vi "ResonatorModulation.vi"(8 "Initial Resonator Voltage":dbl=3.2590378278493897, 9 "Threshold (MHz)":dbl=0.1, 10 "Initial Slow Resonator Voltage":dbl, 11 "f_actual":dbl=394443079.9163828 format="%#_14f") -> (0 "error out":errorcluster, 1 "Slow Resonator Voltage":dbl, 3 "Fast Resonator Voltage":dbl=6.2440401279926325)   [LabVIEW 2017]
uses:
  wlmData.dll
  <vilib>/Analysis/NI_AALBase.lvlib
  <vilib>/Analysis/baseanly.llb/Mean (DBL).vi
  Global M2.vi
panel:
  in  "NUmber Loops":i32=20
  in  "millisecond multiple":u32=1
  in  "DaQ 2":refnum<k21>="M2 Slow Resonator Mod"
  in  "PID gains":T1={"proportional gain (Kc)"=0.05, "integral time (Ti, s)"=0.005, "derivative time (Td, s)"=0.0}
  in  "stop":bool
  in  "DaQ":refnum<k21>="Voltage to M2 Resonator mod"
  out "df/MHz":dbl(graph)=-6.680025041103363
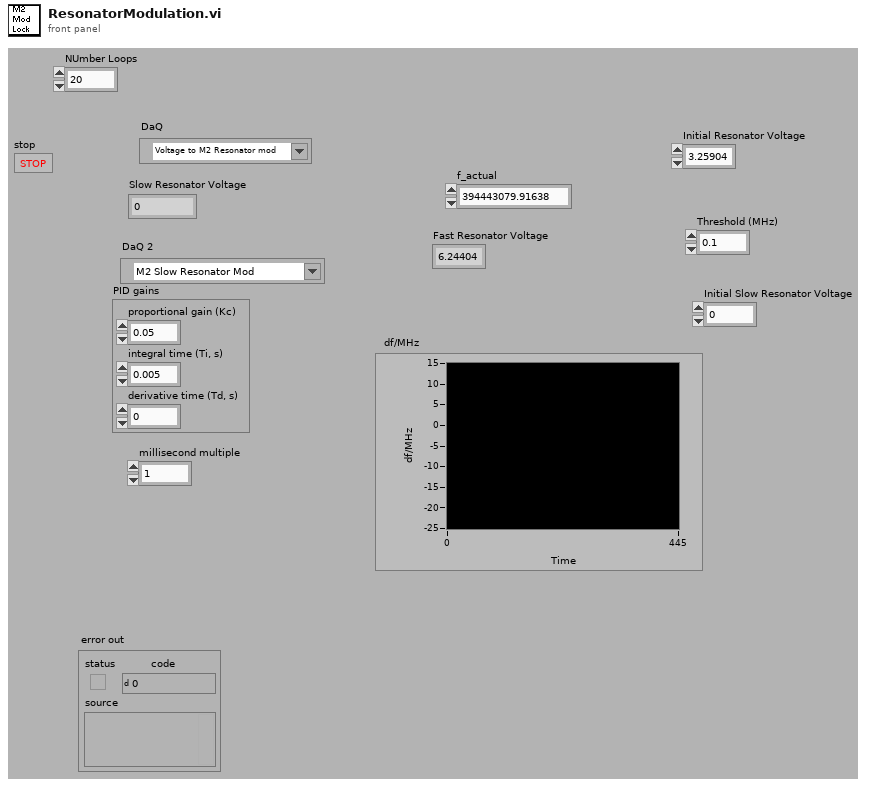
[diagram p1: front panel]
types:
  T1 = cluster{"proportional gain (Kc)":dbl, "integral time (Ti, s)":dbl, "derivative time (Td, s)":dbl}
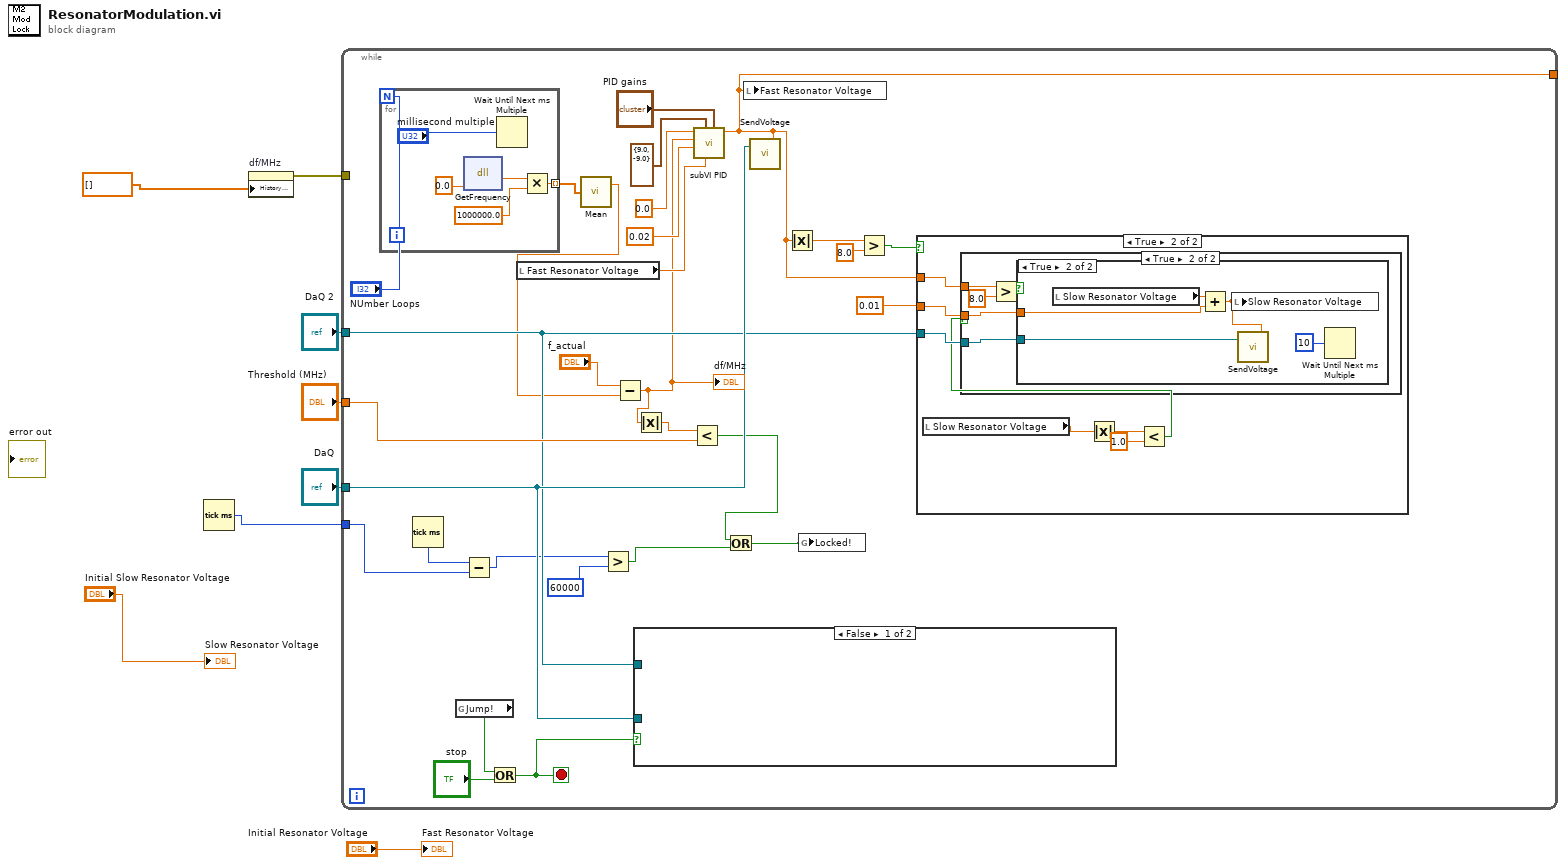
[diagram p0: block diagram]
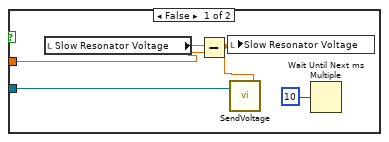
[diagram p4: hidden frame]
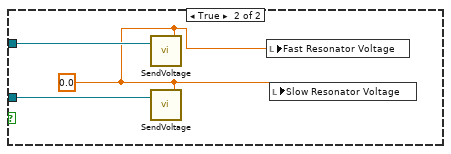
[diagram p5: hidden frame]
diagram:
  n1 = Tick Count (ms)() -> (millisecond timer value=w3:u32)
  n2 = property on="df/MHz" class="WFChart (strict)"("History Data"=dbl[] []) -> (error out=w1:errorcluster)  [unwired: 2 in, 1 out]
  n3 = while {
    tunnel: "DaQ" -> [w32]
    tunnel: [w22] -> _
    tunnel: "DaQ 2" -> [w29]
    tunnel: "Threshold (MHz)" -> [w30]
    tunnel: w3 -> [w20]
    tunnel: w1 -> [_]
    stop <- w27 stop-if-true
    n4 = for {
      N: "NUmber Loops" -> [_]
      tunnel: [w39] -> w14 mode=indexing
      n5 = dll-call lib="wlmData.dll" fn="GetFrequency"("arg1"=0.0) -> ("return type"=w41:dbl)  [unwired: 4 in, 2 out]
      n6 = Wait Until Next ms Multiple(millisecond multiple="millisecond multiple") -> ()  [unwired: 1 out]
      n7 = Multiply(x=w41, y=1000000.0) -> (x*y=w39:dbl)
    }
    n8 = Tick Count (ms)() -> (millisecond timer value=w21:u32)
    n9 = global read "Global M2.vi" "Jump!"() -> (w10:bool)
    n10 = Subtract(x=w21, y=w20) -> (x-y=w19:u32)
    n11 = Or(x=w10, y="stop") -> (x .or. y?=w27:bool)
    n12 = local read "Fast Resonator Voltage"() -> (w31:dbl)
    n13 = call-poly <vilib>:"Mean.vi"("X"=w14) -> ("mean"=w13:dbl)  [unwired: 1 out]
    n14 = Greater?(x=w19, y=u32 60000) -> (0:w17:bool)
    n15 = Subtract(x="f_actual", y=w13) -> (x-y=w12:dbl)
    "df/MHz" <- w12
    n16 = case shown="False" w27 {
      tunnel: w32 -> [_ w67]
      tunnel: w29 -> [_ w66]
      frame False {
      }
      frame True {
        w65 = sgl 0.0 ("value")
        n17 = call "SendVoltage.vi"("value"=w65, "DAQmx Global Channel"=w66) -> ()  [unwired: 1 in, 1 out]
        n18 = call "SendVoltage.vi"("value"=w65, "DAQmx Global Channel"=w67) -> ()  [unwired: 1 in, 1 out]
        n19 = local write "Fast Resonator Voltage"(w65) -> ()
        n20 = local write "Slow Resonator Voltage"(w65) -> ()
      }
    }
    n21 = Absolute Value(x=w12) -> (abs(x)=w11:dbl)
    n22 = Less?(x=w11, y=w30) -> (x < y?=w16:bool)
    n23 = call "subVI PID.vi"("PID gains"="PID gains", "input"=w31, "output range"=cluster{"output high":dbl, "output low":dbl} {"output high"=9.0, "output low"=-9.0}, "dt (s)"=0.02, "process variable"=w12, "setpoint"=0.0) -> ("output"=w22:dbl)  [unwired: 1 in, 4 out]
    n24 = Or(x=w16, y=w17) -> (x .or. y?=w9:bool)
    n25 = local write "Fast Resonator Voltage"(w22) -> ()
    n26 = call "SendVoltage.vi"("value"=w22, "DAQmx Global Channel"=w32) -> ()  [unwired: 1 in, 1 out]
    n27 = Absolute Value(x=w22) -> (abs(x)=w26:dbl)
    n28 = global write "Global M2.vi" "Locked!"(w9) -> ()
    n29 = Greater?(x=w26, y=8.0) -> (0:w24:bool)
    n30 = case shown="True" w24 {
      tunnel: w22 -> [_ w49]
      tunnel: w29 -> [_ w48]
      tunnel: 0.01 ("y") -> [_ w47]
      frame False {
      }
      frame True {
        n31 = local read "Slow Resonator Voltage"() -> (w46:dbl)
        n32 = Absolute Value(x=w46) -> (abs(x)=w45:dbl)
        n33 = Less?(x=w45, y=1.0) -> (x < y?=w43:bool)
        n34 = case shown="True" w43 {
          tunnel: w49 -> [_ w54]
          tunnel: w48 -> [_ w51]
          tunnel: w47 -> [_ w50]
          frame False {
          }
          frame True {
            n35 = Greater?(x=w54, y=8.0) -> (0:w52:bool)
            n36 = case shown="True" w52 {
              tunnel: w51 -> [w59 w63]
              tunnel: w50 -> [w56 w61]
              frame False {
                n37 = local read "Slow Resonator Voltage"() -> (w57:dbl)
                n38 = Subtract(x=w57, y=w56) -> (x-y=w55:dbl)
                n39 = local write "Slow Resonator Voltage"(w55) -> ()
                n40 = call "SendVoltage.vi"("value"=w55, "DAQmx Global Channel"=w59) -> ()  [unwired: 1 in, 1 out]
                n41 = Wait Until Next ms Multiple(millisecond multiple=u32 10) -> ()  [unwired: 1 out]
              }
              frame True {
                n42 = local read "Slow Resonator Voltage"() -> (w64:dbl)
                n43 = Add(x=w64, y=w61) -> (x+y=w62:dbl)
                n44 = local write "Slow Resonator Voltage"(w62) -> ()
                n45 = call "SendVoltage.vi"("value"=w62, "DAQmx Global Channel"=w63) -> ()  [unwired: 1 in, 1 out]
                n46 = Wait Until Next ms Multiple(millisecond multiple=u32 10) -> ()  [unwired: 1 out]
              }
            }
          }
        }
      }
    }
  }
  "Fast Resonator Voltage" <- "Initial Resonator Voltage"
  "Slow Resonator Voltage" <- "Initial Slow Resonator Voltage"
